vi "Untitled 5.vi"() -> ()   [LabVIEW 2009]
panel:
  out "output array":i32[](array[numeric])
  out "Array":i32[][](array[numeric])
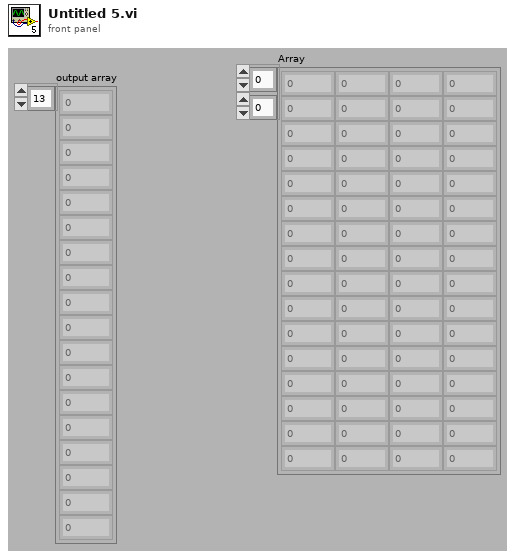
[diagram p1: front panel]
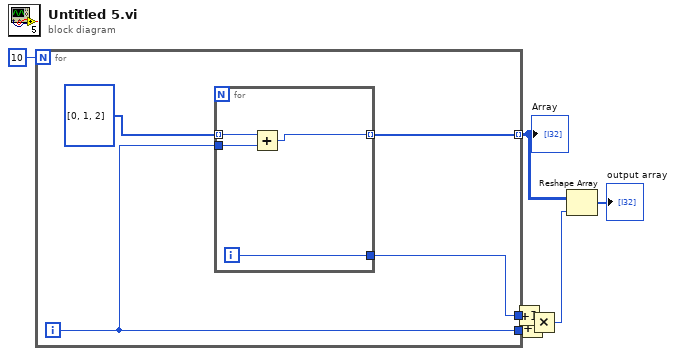
[diagram p0: block diagram]
diagram:
  n1 = for {
    N: 10 -> [_]
    tunnel: [w11] -> w7 mode=indexing
    tunnel: [w9] -> w4
    tunnel: [w10] -> w5
    i -> [w9]
    n2 = for {
      tunnel: i32[] [0, 1, 2] -> [w15] mode=indexing
      tunnel: [w13] -> w11 mode=indexing
      tunnel: [w16] -> w10
      tunnel: w9 -> [w14]
      i -> [w16]
      n3 = Add(x=w15, y=w14) -> (x+y=w13:i32)
    }
  }
  "Array" <- w7
  n4 = Increment(x=w5) -> (x+1=w2:i32)
  n5 = Increment(x=w4) -> (x+1=w1:i32)
  n6 = Multiply(x=w2, y=w1) -> (x*y=w3:i32)
  n7 = Reshape Array(w7, w3) -> (→"output array":i32[])
